vi "py-lv-comm_openConnection.vi"(8 "error in":errorcluster, 11 "TCP address":string="tcp://127.0.0.1:5555") -> (0 "error out":errorcluster, 2 "socket out":refnum<class "zmq_socket.lvclass">, 3 "zmq_context out":refnum<class "zmq_context.lvclass">)   [LabVIEW 2013]
uses:
  <vilib>/addons/zeromq/zmq_context.lvclass
  <vilib>/addons/zeromq/zmq_socket.lvclass
  <vilib>/addons/zeromq/socket_type.ctl
  <vilib>/addons/zeromq/zeromq.lvlib
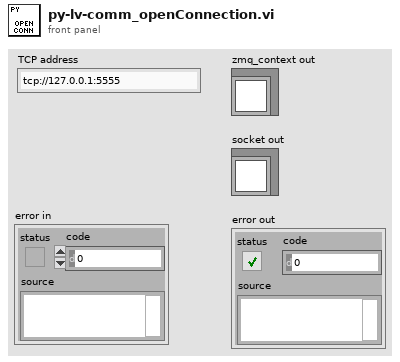
[diagram p1: front panel]
types:
  T1 = typedef "zeromq.lvlib/socket_type.ctl" = enum8{"ZMQ_PAIR", "ZMQ_PUB", "ZMQ_SUB", "ZMQ_REQ", "ZMQ_REP", "ZMQ_DEALER", "ZMQ_ROUTER", "ZMQ_PULL", "ZMQ_PUSH", "ZMQ_XPUB", "ZMQ_XSUB"}
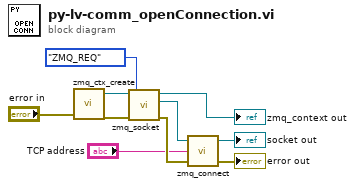
[diagram p0: block diagram]
diagram:
  n1 = call <vilib>:"zmq_ctx_create.vi"("error in"="error in") -> ("error out"=w3:errorcluster, "context out"=w2:refnum<class "zmq_context.lvclass">)  [unwired: 3 in]
  n2 = call <vilib>:"zmq_socket.vi"("error in"=w3, "socket type"=socket_type."ZMQ_REQ", "context in"=w2) -> ("error out"=w7:errorcluster, "socket out"=w6:refnum<class "zmq_socket.lvclass">, "context out"=→"zmq_context out":refnum<class "zmq_context.lvclass">)  [unwired: 2 in]
  n3 = call <vilib>:"zmq_connect.vi"("error in"=w7, "endpoint"="TCP address", "socket in"=w6) -> ("error out"=→"error out":errorcluster, "socket out"=→"socket out":refnum<class "zmq_socket.lvclass">)  [unwired: 1 in]
